vi "TDC_setLftStartInput.vi"(8 "Error In":errorcluster, 11 "Start Channel":i32=1) -> (0 "Error Out":errorcluster)   [LabVIEW 2011]
uses:
  tdcbase.dll
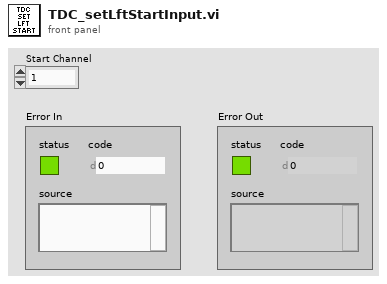
[diagram p1: front panel]
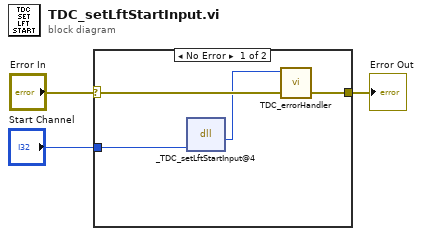
[diagram p0: block diagram]
diagram:
  n1 = case shown="No Error" "Error In" {
    selector: "Error In" -> [w6 w8]
    tunnel: [w5 w8] -> w2
    tunnel: "Start Channel" -> [w7 _]
    frame No Error {
      n2 = dll-call lib="X:/tdcbase.dll" fn="_TDC_setLftStartInput@4"("startChannel"=w7) -> ("return type"=w4:i32)  [unwired: 4 in, 2 out]
      n3 = call "TDC_errorHandler.vi"("Error In"=w6, "TDC Return Code"=w4) -> ("Error Out"=w5:errorcluster)  [unwired: 9 in]
    }
    frame Error {
    }
  }
  "Error Out" <- w2
